vi "Read Configuration (INI) File.vi"(2 "error in (no error)":errorcluster, 3 "configuration file path":path=path "C:/Users/guigue/Documents/hardware/software_config/rga/RGAConfig.ini") -> (0 "error out":errorcluster)   [LabVIEW 2016]
doc: "Illustrates how to read a configuration settings file. Run Write Configuration (INI) File.vi. Then run this VI."
uses:
  <vilib>/Utility/config.llb/Read Key (String).vi
  global/Config_Infos.vi
  <vilib>/Utility/config.llb/Read Key (Double).vi
  <vilib>/Utility/config.llb/NI_LVConfig.lvlib
  <vilib>/Utility/config.llb/Read Key (Path).vi
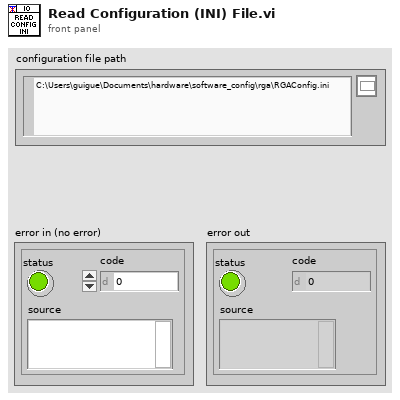
[diagram p1: front panel]
types:
  T1 = typedef "NI_LVConfig.lvlib/Config Data RefNum.ctl" = refnum<k1>
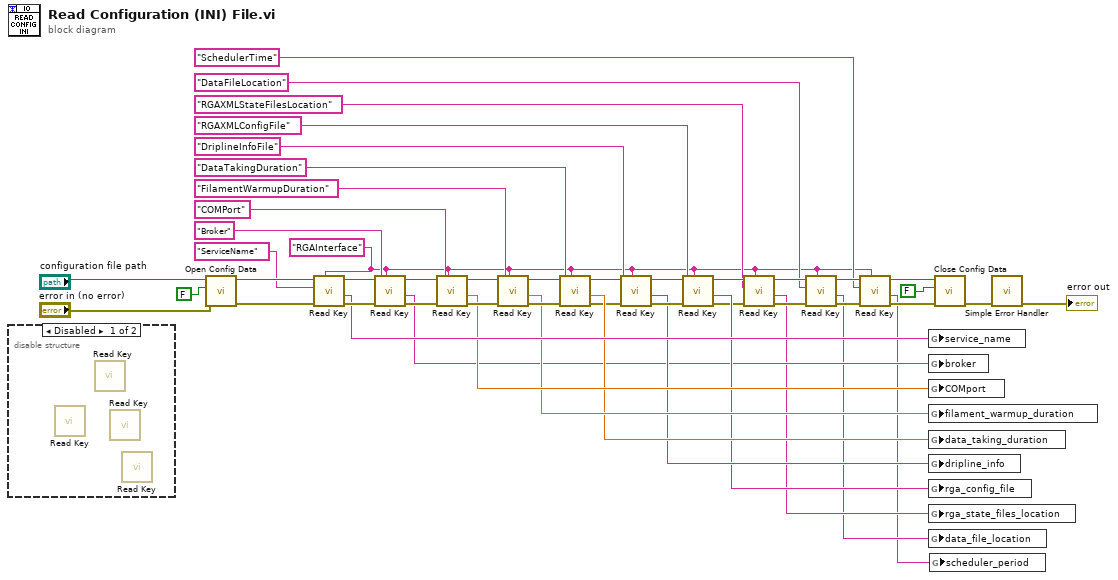
[diagram p0: block diagram]
diagram:
  w2 = "RGAInterface" ("section")
  n1 = disable-structure shown="Disabled" {
    frame Disabled {
      n2 = call-poly <vilib>:"Read Key.vi"() -> ()  [unwired: 6 in, 6 out]
      n3 = call-poly <vilib>:"Read Key.vi"() -> ()  [unwired: 5 in, 7 out]
      n4 = call-poly <vilib>:"Read Key.vi"() -> ()  [unwired: 5 in, 7 out]
      n5 = call-poly <vilib>:"Read Key.vi"() -> ()  [unwired: 6 in, 6 out]
    }
    frame Enabled {
    }
  }
  n6 = call <vilib>:"Open Config Data.vi"("error in (no error)"="error in (no error)", "create file if necessary (T)"=FALSE ("create file if necessary? (T)"), "configuration file path"="configuration file path") -> ("error out"=w45:errorcluster, "refnum"=w47:T1)  [unwired: 6 in, 1 out]
  n7 = call-poly <vilib>:"Read Key.vi"("section"=w2, "error in (no error)"=w45, "key"="ServiceName" ("Key 1"), "refnum"=w47) -> ("error out"=w44:errorcluster, "value"=w43:string, "refnum out"=w42:T1)  [unwired: 2 in, 3 out]
  n8 = call-poly <vilib>:"Read Key.vi"("section"=w2, "error in (no error)"=w44, "key"="Broker" ("Key 2"), "refnum"=w42) -> ("error out"=w39:errorcluster, "value"=w20:string, "refnum out"=w40:T1)  [unwired: 2 in, 3 out]
  n9 = call-poly <vilib>:"Read Key.vi"("section"=w2, "error in (no error)"=w39, "key"="COMPort" ("Key 3"), "refnum"=w40) -> ("error out"=w38:errorcluster, "value"=w37:dbl, "refnum out"=w36:T1)  [unwired: 1 in, 4 out]
  n10 = call-poly <vilib>:"Read Key.vi"("section"=w2, "error in (no error)"=w38, "key"="FilamentWarmupDuration" ("Key 4"), "refnum"=w36) -> ("error out"=w34:errorcluster, "value"=w33:dbl, "refnum out"=w32:T1)  [unwired: 1 in, 4 out]
  n11 = call-poly <vilib>:"Read Key.vi"("section"=w2, "error in (no error)"=w34, "key"="DataTakingDuration" ("Key 5"), "refnum"=w32) -> ("error out"=w27:errorcluster, "value"=w30:dbl, "refnum out"=w28:T1)  [unwired: 1 in, 4 out]
  n12 = call-poly <vilib>:"Read Key.vi"("section"=w2, "error in (no error)"=w27, "key"="DriplineInfoFile" ("Key 5"), "refnum"=w28) -> ("error out"=w25:errorcluster, "value"=w24:string, "refnum out"=w23:T1)  [unwired: 2 in, 3 out]
  n13 = call-poly <vilib>:"Read Key.vi"("section"=w2, "error in (no error)"=w25, "key"="RGAXMLConfigFile" ("Key 5"), "refnum"=w23) -> ("error out"=w17:errorcluster, "value"=w21:string, "refnum out"=w18:T1)  [unwired: 2 in, 3 out]
  n14 = call-poly <vilib>:"Read Key.vi"("section"=w2, "error in (no error)"=w17, "key"="RGAXMLStateFilesLocation" ("Key 5"), "refnum"=w18) -> ("error out"=w12:errorcluster, "value"=w11:string, "refnum out"=w10:T1)  [unwired: 2 in, 3 out]
  n15 = call-poly <vilib>:"Read Key.vi"("section"=w2, "error in (no error)"=w12, "key"="DataFileLocation" ("Key 5"), "refnum"=w10) -> ("error out"=w8:errorcluster, "value"=w7:string, "refnum out"=w6:T1)  [unwired: 2 in, 3 out]
  n16 = call-poly <vilib>:"Read Key.vi"("section"=w2, "error in (no error)"=w8, "key"="SchedulerTime" ("Key 5"), "refnum"=w6) -> ("error out"=w5:errorcluster, "value"=w1:string, "refnum out"=w4:T1)  [unwired: 4 in, 1 out]
  n17 = global write "Config_Infos.vi" "service_name"(w43) -> ()
  n18 = global write "Config_Infos.vi" "broker"(w20) -> ()
  n19 = global write "Config_Infos.vi" "COMport"(w37) -> ()
  n20 = global write "Config_Infos.vi" "filament_warmup_duration"(w33) -> ()
  n21 = global write "Config_Infos.vi" "data_taking_duration"(w30) -> ()
  n22 = global write "Config_Infos.vi" "dripline_info"(w24) -> ()
  n23 = global write "Config_Infos.vi" "rga_config_file"(w21) -> ()
  n24 = global write "Config_Infos.vi" "rga_state_files_location"(w11) -> ()
  n25 = global write "Config_Infos.vi" "data_file_location"(w7) -> ()
  n26 = global write "Config_Infos.vi" "scheduler_period"(w1) -> ()
  n27 = call <vilib>:"Close Config Data.vi"("error in (no error)"=w5, "write file if changed (T)"=FALSE ("write configuration file? (T)"), "refnum"=w4) -> ("error out"=w14:errorcluster)  [unwired: 8 out]
  n28 = call <vilib>:"Simple Error Handler.vi"("error in (no error)"=w14) -> ("error out"=→"error out":errorcluster)  [unwired: 1 in, 7 out]
